vi "Init Events.vi"(8 "error in (no error)":errorcluster, 11 "App in":refnum<class "App.lvclass">) -> (0 "error out":errorcluster, 3 "App out":refnum<class "App.lvclass">)   [LabVIEW 2020, in "PicoG-App.lvlib" / "App.lvclass"]
uses:
  App.lvclass
  App Watcher/App Update Data.ctl
  ViaApp/ViaApp.lvclass
  Builds/picoG/ppl/PicoG-Core.lvlibp/PicoG-Processor/PicoG-Core/DeployPlatform/DeployPlatform.lvclass
  Device/Device.lvclass
  App.lvclass/App.ctl
  App Watcher/App Watcher.lvclass
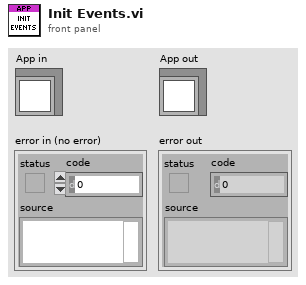
[diagram p1: front panel]
types:
  T1 = typedef "PicoG-App.lvlib/App Watcher.lvclass/App Update Data.ctl" = cluster{"App":refnum<class "ViaApp.lvclass">}
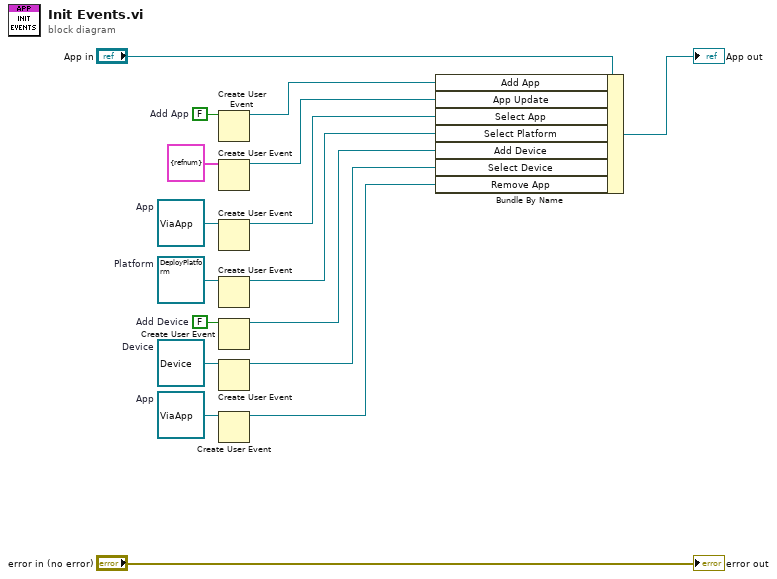
[diagram p0: block diagram]
diagram:
  w2 = refnum<class "ViaApp.lvclass"> refnum  # App
  w4 = refnum<class "Device.lvclass"> refnum  # Device
  w6 = FALSE  # Add Device
  w8 = refnum<class "DeployPlatform.lvclass"> refnum  # Platform
  w10 = refnum<class "ViaApp.lvclass"> refnum  # App
  w14 = FALSE  # Add App
  n1 = Create User Event(user event datatype=w14) -> (user event=w13:refnum<user-event>)  [unwired: 1 in, 1 out]
  n2 = Create User Event(user event datatype=T1 {"App"=refnum} ("App Update Data")) -> (user event=w11:refnum<user-event>)  [unwired: 1 in, 1 out]
  n3 = Create User Event(user event datatype=w10) -> (user event=w9:refnum<user-event>)  [unwired: 1 in, 1 out]
  n4 = Create User Event(user event datatype=w8) -> (user event=w7:refnum<user-event>)  [unwired: 1 in, 1 out]
  n5 = Create User Event(user event datatype=w6) -> (user event=w5:refnum<user-event>)  [unwired: 1 in, 1 out]
  n6 = Create User Event(user event datatype=w4) -> (user event=w3:refnum<user-event>)  [unwired: 1 in, 1 out]
  n7 = Create User Event(user event datatype=w2) -> (user event=w1:refnum<user-event>)  [unwired: 1 in, 1 out]
  n8 = Bundle By Name(cluster="App in", "Add App"=w13, "App Update"=w11, "Select App"=w9, "Select Platform"=w7, "Add Device"=w5, "Select Device"=w3, "Remove App"=w1) -> (→"App out":refnum<class "App.lvclass">)
  "error out" <- "error in (no error)"
